vi "SRTS_Resp_Save2.vi"(7 "XLS ref.":refnum<vi>, 8 "error in":errorcluster, 10 "Resp Results":T1 {"R3AOM_RespT" format="%#.3f"; "R3DOM_RespT" format="%#.3f"; "R3AOM_TS" format="%#.3f"; "R3DOM_TS" format="%#.3f"; "RIM3_TS" format="%#.3f"; "R2AOM_RespT" format="%#.3f"; "R2DOM_RespT" format="%#.3f"; "R2AOM_TS" format="%#.3f"; "R2DOM_TS" format="%#.3f"; "RIM2_TS" format="%#.3f"; "R1AOM_RespT" format="%#.3f"; "R1DOM_RespT" format="%#.3f"; "R1AOM_TS" format="%#.3f"; "R1DOM_TS" format="%#.3f"; "RIM1_TS" format="%#.3f"; "TAOM_RespT" format="%#.3f"; "TDOM_RespT" format="%#.3f"; "TAOM_TS" format="%#.3f"; "TDOM_TS" format="%#.3f"; "TIM_TS" format="%#.3f"; "WAOM_RespT" format="%#.3f"; "WDOM_RespT" format="%#.3f"; "WAOM_TS" format="%#.3f"; "WDOM_TS" format="%#.3f"; "WAIM_TS" format="%#.3f"}, 11 "XLS in":refnum<class "XLS.lvclass">=refnum) -> (0 "error out":errorcluster, 2 "Progress":i32, 3 "XLS out":refnum<class "XLS.lvclass">)   [LabVIEW 2017, in "Report_lib.lvlib" / "XLS.lvclass"]
uses:
  XLS.lvclass
  TypeDefs/RespT_Results.ctl
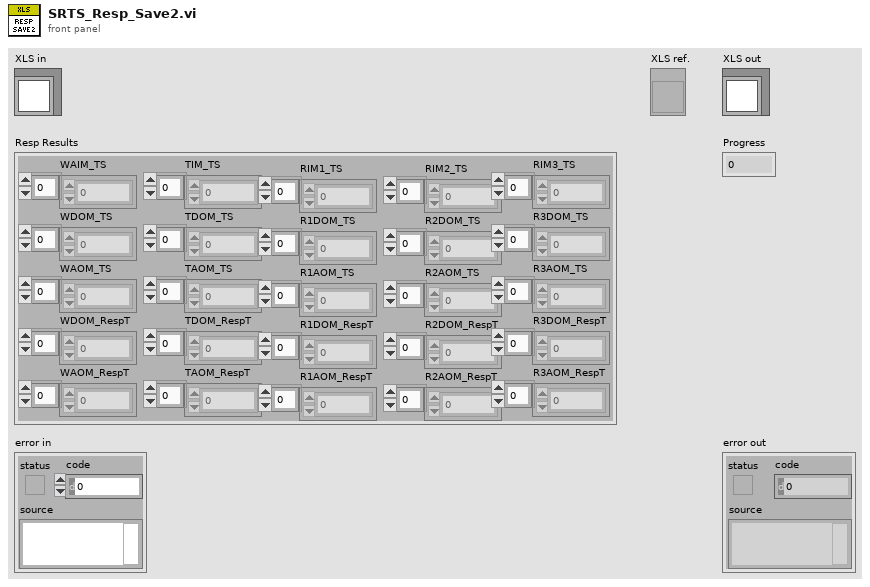
[diagram p1: front panel]
types:
  T1 = typedef "RespT_Results.ctl" = cluster{"WAIM_TS":dbl[], "WDOM_TS":dbl[], "WAOM_TS":dbl[], "WDOM_RespT":dbl[], "WAOM_RespT":dbl[], "TIM_TS":dbl[], "TDOM_TS":dbl[], "TAOM_TS":dbl[], "TDOM_RespT":dbl[], "TAOM_RespT":dbl[], "RIM1_TS":dbl[], "R1DOM_TS":dbl[], "R1AOM_TS":dbl[], "R1DOM_RespT":dbl[], "R1AOM_RespT":dbl[], "RIM2_TS":dbl[], "R2DOM_TS":dbl[], "R2AOM_TS":dbl[], "R2DOM_RespT":dbl[], "R2AOM_RespT":dbl[], "RIM3_TS":dbl[], "R3DOM_TS":dbl[], "R3AOM_TS":dbl[], "R3DOM_RespT":dbl[], "R3AOM_RespT":dbl[]}
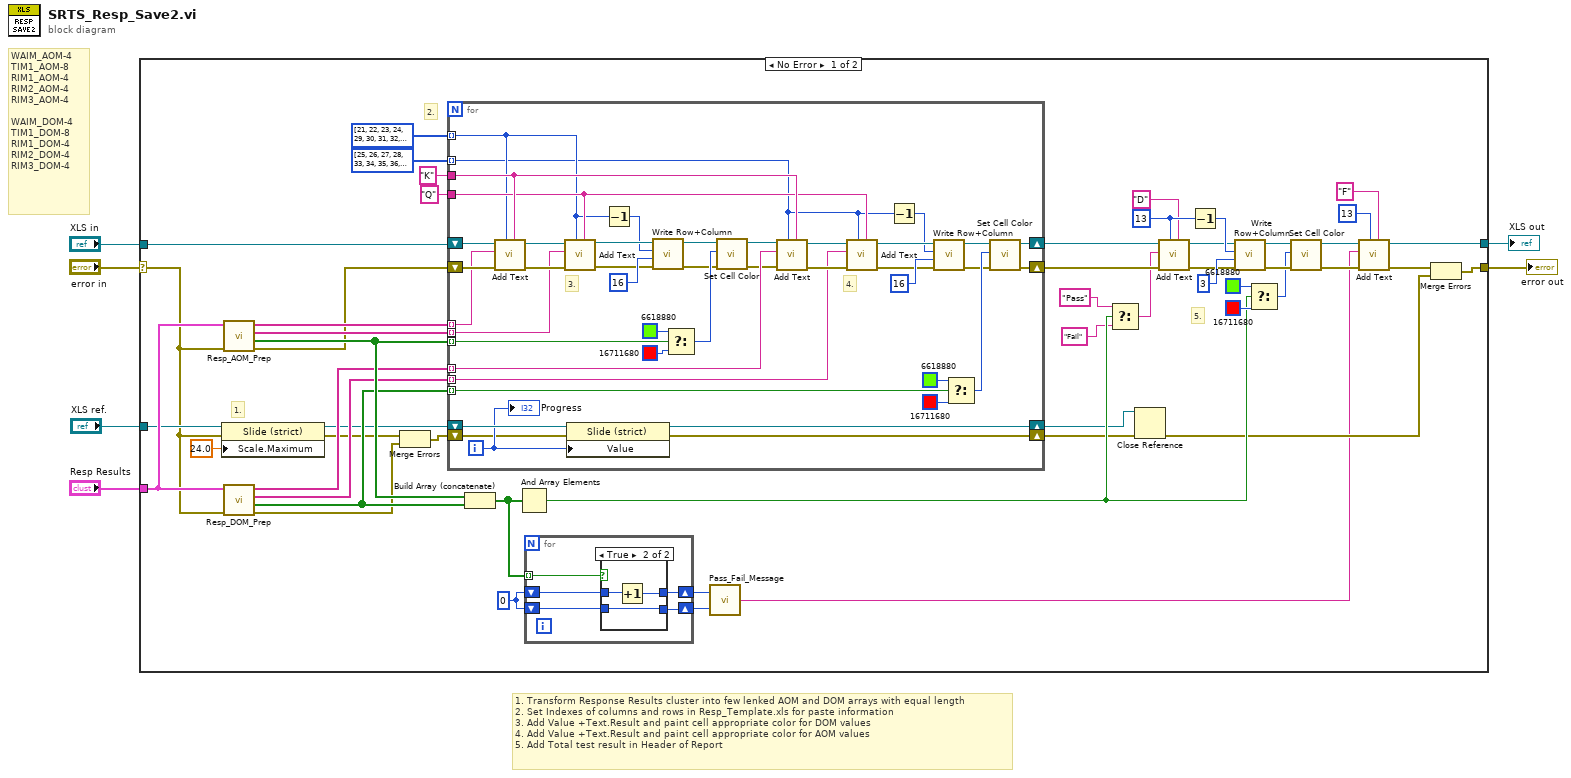
[diagram p0: block diagram]
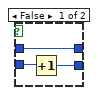
[diagram p2: hidden frame]
diagram:
  # "1. Transform Response Results cluster into few lenked AOM and DOM arrays with equal length\n2. Set Indexes of columns and rows in Resp_Template.xls for paste information\n3. Add Value +Text.Result and paint cell appropriate color for DOM values\n4. Add Value +Text.Result and paint cell appropriate color for AOM values\n5. Add Total test result in Header of Report"
  # "WAIM_AOM-4\nTIM1_AOM-8\nRIM1_AOM-4\nRIM2_AOM-4\nRIM3_AOM-4\n\nWAIM_DOM-4\nTIM1_DOM-8\nRIM1_DOM-4\nRIM2_DOM-4\nRIM3_DOM-4"
  n1 = case shown="No Error" "error in" {
    selector: "error in" -> [w22 w114]
    tunnel: [w58 w114] -> w5
    tunnel: [w11 w113] -> w3
    tunnel: "XLS in" -> [w53 w113]
    tunnel: "Resp Results" -> [w33 _]
    tunnel: "XLS ref." -> [w25 _]
    frame No Error {
      w18 = 0
      w37 = 13 ("Index")
      # "5."
      # "2."
      # "1."
      n2 = property class="Slide (strict)"(reference=w25, error in=w22, "Scale.Maximum"=24.0 ("Scale.Range:Maximum")) -> (reference out=w24:refnum<vi>, error out=w21:errorcluster)
      n3 = call "Resp_AOM_Prep.vi"("error in"=w22, "Resp_Result"=w33) -> ("error out"=w29:errorcluster, "Result_Bool"=w36:bool[], "Result_str"=w35:string[], "Value_str"=w34:string[])  [unwired: 6 in]
      n4 = call "Resp_DOM_Prep.vi"("error in"=w22, "Resp_Result"=w33) -> ("error out"=w20:errorcluster, "Result_Bool"=w30:bool[], "Result_str"=w31:string[], "Value_str"=w32:string[])  [unwired: 6 in]
      n5 = Merge Errors(w21, w20) -> (w19:errorcluster)
      n6 = for {
        tunnel: i32[] [21, 22, 23, 24, 29, 30, 31, 32, 37, 38, 39, 40, 45, 46, 47, 48, 53, 54, 55, 56, 61, 62, 63, 64] ("AOM_indexies") -> [w78] mode=indexing
        tunnel: i32[] [25, 26, 27, 28, 33, 34, 35, 36, 41, 42, 43, 44, 49, 50, 51, 52, 57, 58, 59, 60, 65, 66, 67, 68] ("DOM_indexies") -> [w76] mode=indexing
        tunnel: "K" -> [w112]
        tunnel: "Q" -> [w111]
        shift-right: [w80] -> w52
        shift-left: w53 -> [w106]
        shift-right: [w81] -> w51
        shift-left: w29 -> [w105]
        tunnel: w34 -> [w104] mode=indexing
        tunnel: w35 -> [w103] mode=indexing
        tunnel: w32 -> [w102] mode=indexing
        tunnel: w31 -> [w101] mode=indexing
        tunnel: w36 -> [w90] mode=indexing
        tunnel: w30 -> [w79] mode=indexing
        shift-right: [w72] -> w28
        shift-left: w24 -> [w74]
        shift-right: [w70] -> w27
        shift-left: w19 -> [w71]
        i -> [w73]
        # "4."
        # "3."
        n7 = call "Add Text.vi"("Adr"=w112, "Index"=w78, "error in"=w105, "text"=w104, "XLS in"=w106) -> ("error out"=w108:errorcluster, "XLS out"=w110:refnum<class "XLS.lvclass">)  [unwired: 5 in]
        n8 = call "Add Text.vi"("Adr"=w111, "Index"=w78, "error in"=w108, "text"=w103, "XLS in"=w110) -> ("error out"=w94:errorcluster, "XLS out"=w93:refnum<class "XLS.lvclass">)  [unwired: 5 in]
        n9 = property class="Slide (strict)"(reference=w74, error in=w71, "Value"=w73) -> (reference out=w72:refnum<vi>, error out=w70:errorcluster)
        n10 = Decrement(x=w78) -> (x-1=w77:i32)
        n11 = call "Write Row+Column.vi"("error in"=w94, "column"=16, "row"=w77, "XLS in"=w93) -> ("error out"=w98:errorcluster, "XLS out"=w97:refnum<class "XLS.lvclass">)  [unwired: 6 in]
        n12 = Select(t=u32 6618880, s=w90, f=u32 16711680) -> (s? t:f=w99:u32)
        n13 = call "Set Cell Color.vi"("error in"=w98, "color"=w99, "XLS in"=w97) -> ("error out"=w91:errorcluster, "XLS out"=w92:refnum<class "XLS.lvclass">)  [unwired: 7 in]
        n14 = call "Add Text.vi"("Adr"=w112, "Index"=w76, "error in"=w91, "text"=w102, "XLS in"=w92) -> ("error out"=w107:errorcluster, "XLS out"=w109:refnum<class "XLS.lvclass">)  [unwired: 5 in]
        n15 = call "Add Text.vi"("Adr"=w111, "Index"=w76, "error in"=w107, "text"=w101, "XLS in"=w109) -> ("error out"=w83:errorcluster, "XLS out"=w82:refnum<class "XLS.lvclass">)  [unwired: 5 in]
        n16 = Decrement(x=w76) -> (x-1=w75:i32)
        n17 = call "Write Row+Column.vi"("error in"=w83, "column"=16, "row"=w75, "XLS in"=w82) -> ("error out"=w88:errorcluster, "XLS out"=w87:refnum<class "XLS.lvclass">)  [unwired: 6 in]
        n18 = Select(t=u32 6618880, s=w79, f=u32 16711680) -> (s? t:f=w89:u32)
        n19 = call "Set Cell Color.vi"("error in"=w88, "color"=w89, "XLS in"=w87) -> ("error out"=w81:errorcluster, "XLS out"=w80:refnum<class "XLS.lvclass">)  [unwired: 7 in]
        "Progress" <- w73
      }
      n20 = Build Array (concatenate)(w36, w30) -> (w17:bool[])
      n21 = And Array Elements(Boolean array=w17) -> (logical AND=w41:bool)
      n22 = for {
        tunnel: w17 -> [w63] mode=indexing
        shift-right: [w59] -> w16
        shift-left: w18 -> [w62]
        shift-right: [w60] -> w15
        shift-left: w18 -> [w61]
        n23 = case shown="True" w63 {
          tunnel: w62 -> [w64 w68]
          tunnel: w61 -> [w66 w69]
          tunnel: [w65 w69] -> w60
          tunnel: [w64 w67] -> w59
          frame False {
            n24 = Increment(x=w66) -> (x+1=w65:i32)
          }
          frame True {
            n25 = Increment(x=w68) -> (x+1=w67:i32)
          }
        }
      }
      n26 = call "Pass_Fail_Message.vi"("Failed"=w15, "Passed"=w16) -> ("Result Message"=w10:string)
      n27 = Select(t="Pass" ("Adr"), s=w41, f="Fail" ("Adr")) -> (s? t:f=w38:string)
      n28 = Close Reference(reference=w28, error in (no error)=w27) -> (error out=w26:errorcluster)
      n29 = call "Add Text.vi"("Adr"="D", "Index"=w37, "error in"=w51, "text"=w38, "XLS in"=w52) -> ("error out"=w42:errorcluster, "XLS out"=w43:refnum<class "XLS.lvclass">)  [unwired: 5 in]
      n30 = Decrement(x=w37) -> (x-1=w50:i32)
      n31 = call "Write Row+Column.vi"("error in"=w42, "column"=3, "row"=w50, "XLS in"=w43) -> ("error out"=w47:errorcluster, "XLS out"=w48:refnum<class "XLS.lvclass">)  [unwired: 6 in]
      n32 = Select(t=u32 6618880, s=w41, f=u32 16711680) -> (s? t:f=w44:u32)
      n33 = call "Set Cell Color.vi"("error in"=w47, "color"=w44, "XLS in"=w48) -> ("error out"=w14:errorcluster, "XLS out"=w13:refnum<class "XLS.lvclass">)  [unwired: 7 in]
      n34 = call "Add Text.vi"("Adr"="F", "Index"=13, "error in"=w14, "text"=w10, "XLS in"=w13) -> ("error out"=w12:errorcluster, "XLS out"=w11:refnum<class "XLS.lvclass">)  [unwired: 5 in]
      n35 = Merge Errors(w12, w26) -> (w58:errorcluster)
    }
    frame Error {
    }
  }
  "error out" <- w5
  "XLS out" <- w3
